vi "Get Left.vi"(8 "error in (no error)":errorcluster, 11 "SnailNum in":refnum<class "SnailNum.lvclass">) -> (0 "error out":errorcluster, 2 "Left":refnum<class "SnailNum.lvclass">, 3 "SnailNum out":refnum<class "SnailNum.lvclass">)   [LabVIEW 2020, in "SnailNum.lvclass"]
uses:
  SnailNum.lvclass
  SnailNum.lvclass/SnailNum.ctl
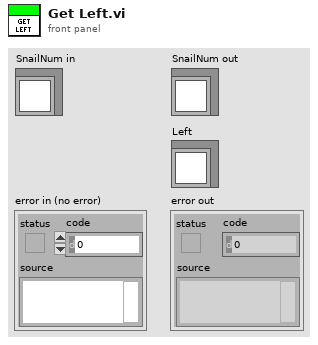
[diagram p1: front panel]
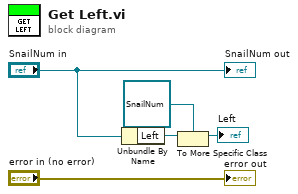
[diagram p0: block diagram]
diagram:
  n1 = Unbundle By Name("SnailNum in") -> ("Left"=w3:refnum<class "SnailElement.lvclass">)
  n2 = To More Specific Class(target class=refnum<class "SnailNum.lvclass"> refnum ("SnailNum.lvclass"), reference=w3) -> (specific class reference=→"Left":refnum<class "SnailNum.lvclass">)  [unwired: 1 in, 1 out]
  "error out" <- "error in (no error)"
  "SnailNum out" <- "SnailNum in"
